vi "生成任意波形.vi"(9 "限流":dbl, 10 "采样点":dbl=1e-05, 11 "波形描述":string[][](table)) -> (3 "波形图":waveform(dbl))   [LabVIEW 2020, in "功能选择.xctl"]
uses:
  <vilib>/measure/maresamp.llb/Resample Waveform (continuous).vi
  <vilib>/measure/NI_MAPro.lvlib
panel:
  # "L=线性\nlog=对数\nP=脉冲\nS=阶跃"
  # "类型为对数时备注为渐近线线\n脉冲时为占空比0-99.9\n阶跃信号为突变位置0-100"
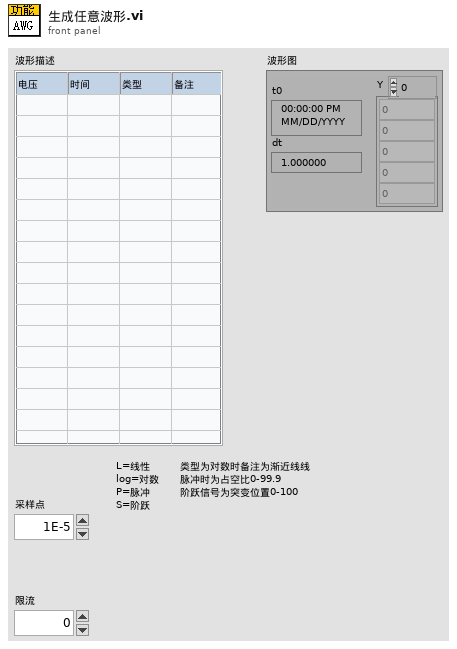
[diagram p1: front panel]
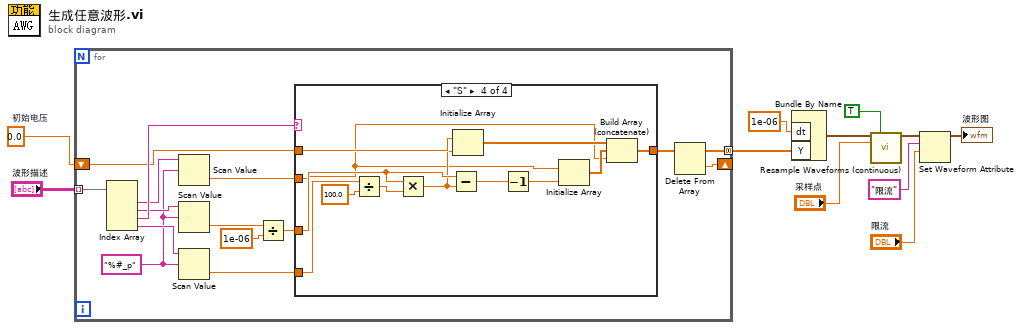
[diagram p0: block diagram]
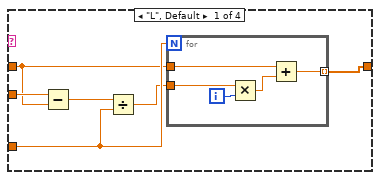
[diagram p2: hidden frame]
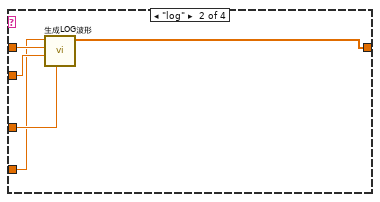
[diagram p3: hidden frame]
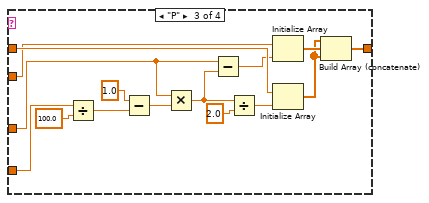
[diagram p4: hidden frame]
diagram:
  w10 = 0.0  # 初始电压
  n1 = for {
    tunnel: "波形描述" -> [w26] mode=indexing
    shift-right: [w16] -> _
    shift-left: w10 -> [w24]
    tunnel: [w14] -> w9 mode=concatenating
    w12 = "%#_p" ("格式字符串")
    n2 = Index Array(array=w26) -> (element #1=w22:string, element #2=w23:string, element #3=w25:string, element #4=w21:string)  [unwired: 4 in]
    n3 = Scan Value(string=w22, format string=w12) -> (value=w20:dbl)  [unwired: 1 in, 1 out]
    n4 = Scan Value(string=w23, format string=w12) -> (value=w19:dbl)  [unwired: 1 in, 1 out]
    n5 = Scan Value(string=w21, format string=w12) -> (value=w15:dbl)  [unwired: 1 in, 1 out]
    n6 = Divide(x=w19, y=1e-06) -> (x/y=w13:dbl)
    n7 = case shown="\"S\"" w25 {
      tunnel: w24 -> [w27 w42 w57 w69]
      tunnel: w20 -> [w29 w41 w52 w59]
      tunnel: w13 -> [w31 w40 w50 w62]
      tunnel: [w28 w38 w47 w66] -> w17
      tunnel: w15 -> [_ w39 w56 w64]
      frame "L", Default {
        n8 = Subtract(x=w29, y=w27) -> (x-y=w32:dbl)
        n9 = Divide(x=w32, y=w31) -> (x/y=w30:dbl)
        n10 = for {
          N: w31 -> [_]
          tunnel: w30 -> [w37]
          tunnel: w27 -> [w35]
          tunnel: [w33] -> w28 mode=indexing
          i -> [w36]
          n11 = Multiply(x=w37, y=w36) -> (x*y=w34:dbl)
          n12 = Add(x=w35, y=w34) -> (x+y=w33:dbl)
        }
      }
      frame "log" {
        n13 = call "生成LOG波形.vi"("采样"=w40, "end"=w41, "start"=w42, "渐近线"=w39) -> ("波形"=w38:dbl[])  [unwired: 7 in]
      }
      frame "P" {
        n14 = Divide(x=w56, y=100.0) -> (x/y=w54:dbl)
        n15 = Subtract(x=1.0, y=w54) -> (x-y=w51:dbl)
        n16 = Multiply(x=w50, y=w51) -> (x*y=w46:dbl)
        n17 = Subtract(x=w50, y=w46) -> (x-y=w49:dbl)
        n18 = Divide(x=w46, y=2.0) -> (x/y=w44:dbl)
        n19 = Initialize Array(w52, w49) -> (w48:dbl[])
        n20 = Initialize Array(w57, w44) -> (w43:dbl[])
        n21 = Build Array (concatenate)(w43, w48, w43) -> (w47:dbl[])
      }
      frame "S" {
        n22 = Divide(x=w64, y=100.0) -> (x/y=w63:dbl)
        n23 = Multiply(x=w62, y=w63) -> (x*y=w60:dbl)
        n24 = Subtract(x=w62, y=w60) -> (x-y=w61:dbl)
        n25 = Initialize Array(w69, w60) -> (w68:dbl[])
        n26 = Decrement(x=w61) -> (x-1=w58:dbl)
        n27 = Initialize Array(w59, w58) -> (w67:dbl[])
        n28 = Build Array (concatenate)(w68, w67, w59) -> (w66:dbl[])
      }
    }
    n29 = Delete From Array(array=w17) -> (deleted portion=w16:dbl, array with subset deleted=w14:dbl[])  [unwired: 2 in]
  }
  n30 = Bundle By Name("dt"=1e-06 ("y"), "Y"=w9) -> (w6:waveform(dbl))  [unwired: 1 in]
  n31 = call-poly <vilib>:"Resample Waveforms (continuous).vi"("waveform in"=w6, "reset"=TRUE, "dt"="采样点") -> ("resampled waveform out"=w5:waveform(dbl))  [unwired: 8 in, 4 out]
  n32 = Set Waveform Attribute(5:"限流", 6:"限流" ("名称"), 7:w5) -> (3:→"波形图":waveform(dbl))  [unwired: 1 in, 2 out]
